vi "BME_DG_LoadAllCardParameters.vi"(8 "error in (no error)":errorcluster, 9 "TimeList":bool, 10 "ModuloCounter":bool, 11 "EventCounter":bool) -> (0 "error out":errorcluster)   [LabVIEW 2009, in "POLARIS BME DG.lvlib"]
uses:
  POLARIS BME DG.lvlib
  BME DLL/DelayGenerator.dll
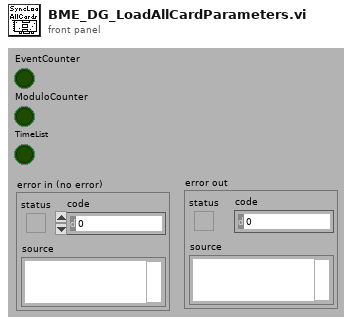
[diagram p1: front panel]
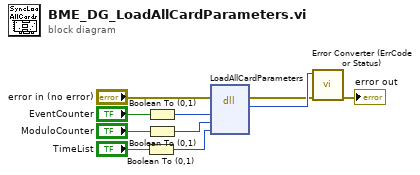
[diagram p0: block diagram]
diagram:
  n1 = Boolean To (0,1)(Boolean="TimeList") -> (0, 1=w1:i16)
  n2 = Boolean To (0,1)(Boolean="EventCounter") -> (0, 1=w3:i16)
  n3 = Boolean To (0,1)(Boolean="ModuloCounter") -> (0, 1=w2:i16)
  n4 = dll-call lib="C:/CS Framework/LVSCC/LV2009/GPL/Projects/cs-framework/CSClass/CSPOLARIS/POLARIS BME DG/BME DLL/DelayGenerator.dll" fn="LoadAllCardParameters" label="Activate_DG_BME"(error in="error in (no error)", "bEventCounter"=w3, "bModuloCounter"=w2, "bTimeList"=w1) -> (error out=w8:errorcluster, "return type"=w9:i32)  [unwired: 5 in, 1 out]
  n5 = call "Error Converter (ErrCode or Status).vi"("error in (no error)"=w8, "error code"=w9) -> ("error out"=→"error out":errorcluster)  [unwired: 9 in]
